vi "read_Shapes.vi"() -> ()   [LabVIEW 2019]
uses:
  Program Files (x86)/National Instruments/LabVIEW 2019/examples/RTI DDS Toolkit/ShapesDemo/support/RTI Connext DDS Shape Type.ctl
  <vilib>/RTI DDS Toolkit/Types/DDS Sample Info.ctl
  <vilib>/RTI DDS Toolkit/Types/RTI DDS Advanced Reader Configuration.ctl
  <vilib>/RTI DDS Toolkit/Library/LVDDS_library.lvlib
panel:
  in  "Tab Control":enum32{"Main", "config"}(tab)
  out "DDS Data":string[][](table)=[["RED", "203", "241", " 30"]]
  in  "Query condition":string
  out "Sample Info":T1={"DDS_SampleStateKind"=enum."DDS_NOT_READ_SAMPLE_STATE", "DDS_ViewStateKind"=enum."DDS_NOT_NEW_VIEW_STATE", "DDS_InstanceStateKind"=enum."DDS_ALIVE_INSTANCE_STATE", "sec"=1653553695, "nanosec"=521993280, "valid_data"=TRUE}
  out "XY Graph":cluster{"Y":dbl[], "Y":dbl[]}[](graph)=[{"Y"=[203.0], "Y"=[241.0]}]
  out "shapesize":i32(slide)=30 scale=0.0..100.0
  in  "Enter a shape 'color' to see the square moving in 'XY Graph' and its size in 'shapesize'":string="RED"
  in  "Enable DDS":bool=TRUE
  in  "Stop":bool
  in  "Type Name":string="ShapeType"
  in  "Key Name":string="color"
  in  "Topic Name":string="Circle"
  in  "Advanced Reader Configuration":T2
  in  "error in (no error)":errorcluster
  in  "ShapeType 2":T3
  out "error out":errorcluster
  out "ShapeType":T3={"color"="RED", "x"=203, "y"=241, "shapesize"=30}
  # "RTI DDS Read shape"
  # "Source Timestamp"
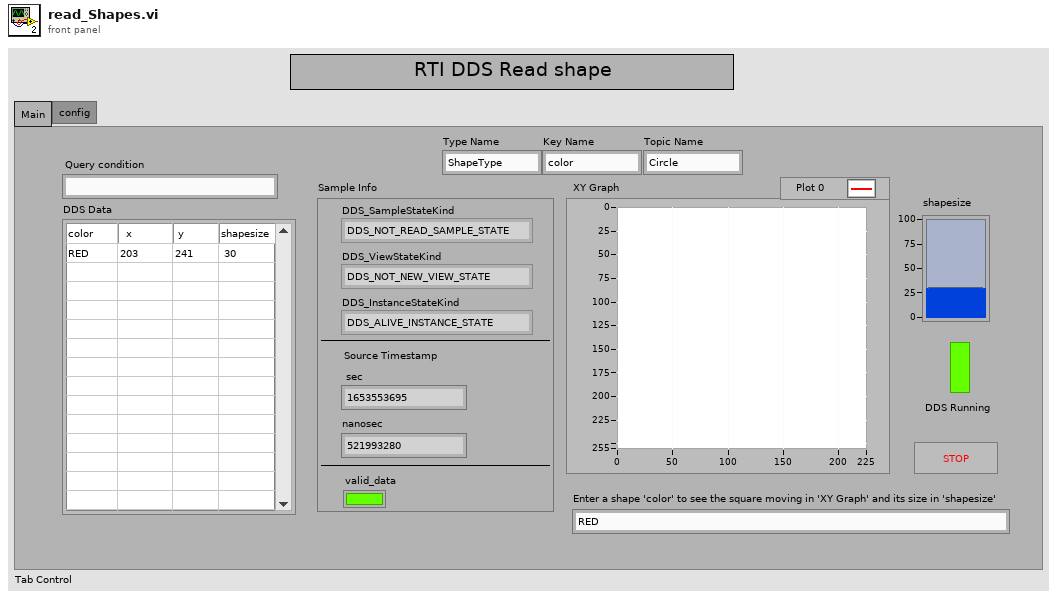
[diagram p1: front panel]
types:
  T1 = typedef "LVDDS_library.lvlib/DDS Sample Info.ctl" = cluster{"DDS_SampleStateKind":enum32{"DDS_INVALID_SAMPLE_STATE", "DDS_READ_SAMPLE_STATE", "DDS_NOT_READ_SAMPLE_STATE"}, "DDS_ViewStateKind":enum32{"DDS_INVALID_SAMPLE_STATE", "DDS_NEW_VIEW_STATE", "DDS_NOT_NEW_VIEW_STATE"}, "DDS_InstanceStateKind":enum32{"DDS_INVALID_STATE", "DDS_ALIVE_INSTANCE_STATE", "DDS_NOT_ALIVE_DISPOSED_INSTANCE_STATE", "", "DDS_NOT_ALIVE_NO_WRITERS_INSTANCE_STATE"}, "sec":i32, "nanosec":u32, "valid_data":bool}
  T2 = typedef "LVDDS_library.lvlib/RTI DDS Advanced Reader Configuration.ctl" = cluster{"typeName":string, "keyName":string, "domainParticipantQoSProfile":string, "dataReaderQoSProfile":string, "forceArrayMapping?":bool, "forceExclusiveReader?":bool, "forceRead? (only ExclusiveReader)":bool, "forceUnboundedString?":bool}
  T3 = typedef "RTI Connext DDS Shape Type.ctl" = cluster{"color":string, "x":i32, "y":i32, "shapesize":i32}
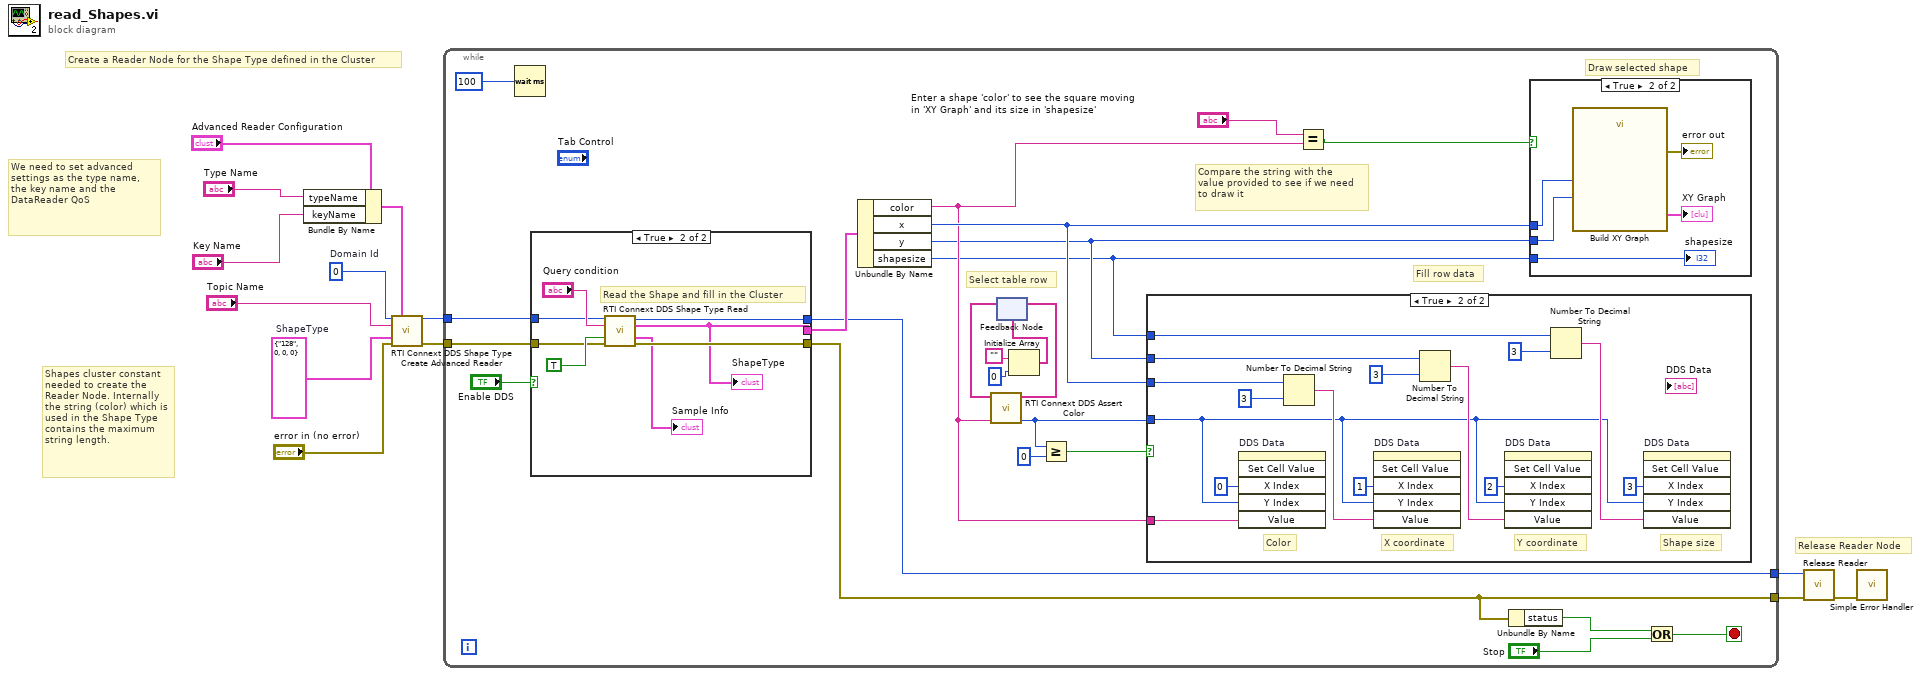
[diagram p0: block diagram]
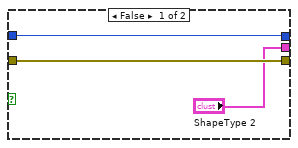
[diagram p3: hidden frame]
diagram:
  w7 = T3 {"color"="128", "x"=0, "y"=0, "shapesize"=0}  # ShapeType
  w2 = u32 0  # Domain Id
  # "We need to set advanced settings as the type name,\nthe key name and the DataReader QoS"
  # "Release Reader Node"
  # "Shapes cluster constant needed to create the Reader Node. Internally the string (color) which is used in the Shape Type contains the maximum string length."
  # "Create a Reader Node for the Shape Type defined in the Cluster"
  n1 = Bundle By Name(cluster="Advanced Reader Configuration", "typeName"="Type Name", "keyName"="Key Name") -> (w6:T2)
  n2 = call "RTI Connext DDS Shape Type Create Advanced Reader.vi"("Domain Id"=w2, "Advanced Reader Configuration"=w6, "Topic Name"="Topic Name", "MyComplexType type"=w7, "error in (no error)"="error in (no error)") -> ("DDS Object Ref"=w1:u64, "error out"=w5:errorcluster)  [unwired: 9 in]
  n3 = while {
    tunnel: [w15] -> w13
    tunnel: w5 -> [w21]
    tunnel: [w20] -> w4
    tunnel: w1 -> [w14]
    stop <- w26 stop-if-true
    # "Compare the string with the\nvalue provided to see if we need\nto draw it"
    # "Select table row"
    # "Draw selected shape"
    # "Fill row data"
    n4 = Wait (ms)(milliseconds to wait=u32 100) -> ()  [unwired: 1 out]
    n5 = case shown="True" "Enable DDS" {
      tunnel: ["ShapeType 2" w56] -> w36
      tunnel: w14 -> [w55 w59]
      tunnel: w21 -> [w54 w58]
      tunnel: [w55 w57] -> w15
      tunnel: [w54 w63] -> w20
      frame False {
      }
      frame True {
        # "Read the Shape and fill in the Cluster"
        n6 = call "RTI Connext DDS Shape Type Read.vi"("DDS Object Ref in"=w59, "Query Condition"="Query condition", "Only New Samples"=TRUE, "error in (no error)"=w58) -> ("DDS Object Ref out"=w57:u64, "Read Sample"=w56:T3, "DDS Sample Info"=→"Sample Info":T1, "error out"=w63:errorcluster)  [unwired: 7 in, 1 out]
        "ShapeType" <- w56
      }
    }
    n7 = Unbundle By Name(w36) -> ("color"=w22:string, "x"=w37:i32, "y"=w17:i32, "shapesize"=w16:i32)
    n8 = Initialize Array("", 0 ("dimension size")) -> (w33:string[])
    n9 = feedback #1(w33) -> (w28:string[])
    n10 = call "RTI Connext DDS Assert Color.vi"("Color"=w22, "Input Array"=w28) -> ("Position"=w18:i32, "Output Array"=w29:string[])  [unwired: 8 in]
    n11 = feedback-in #1(w29) -> ()
    n12 = Greater Or Equal?(x=w18, y=0) -> (x >= y?=w32:bool)
    n13 = case shown="True" w32 {
      tunnel: w37 -> [_ w51]
      tunnel: w17 -> [_ w50]
      tunnel: w18 -> [_ w39]
      tunnel: w22 -> [_ w46]
      tunnel: w16 -> [_ w49]
      frame False {
      }
      frame True {
        # "Shape size"
        # "Y coordinate"
        # "X coordinate"
        # "Color"
        n14 = invoke on="DDS Data" class="Tbl (strict)" method="Set Cell Value"("X Index"=0, "Y Index"=w39, "Value"=w46) -> ()  [unwired: 3 in, 6 out]
        n15 = Number To Decimal String(number=w51, width (-)=3) -> (decimal integer string=w43:string)
        n16 = invoke on="DDS Data" class="Tbl (strict)" method="Set Cell Value"("X Index"=1, "Y Index"=w39, "Value"=w43) -> ()  [unwired: 3 in, 6 out]
        n17 = Number To Decimal String(number=w50, width (-)=3) -> (decimal integer string=w42:string)
        n18 = invoke on="DDS Data" class="Tbl (strict)" method="Set Cell Value"("X Index"=2, "Y Index"=w39, "Value"=w42) -> ()  [unwired: 3 in, 6 out]
        n19 = Number To Decimal String(number=w49, width (-)=3) -> (decimal integer string=w40:string)
        n20 = invoke on="DDS Data" class="Tbl (strict)" method="Set Cell Value"("X Index"=3, "Y Index"=w39, "Value"=w40) -> ()  [unwired: 3 in, 6 out]
      }
    }
    n21 = Equal?(x="Enter a shape 'color' to see the square moving in 'XY Graph' and its size in 'shapesize'", y=w22) -> (x = y?=w24:bool)
    n22 = Unbundle By Name(w20) -> ("status"=w19:bool)
    n23 = case shown="True" w24 {
      tunnel: w37 -> [_ w65]
      tunnel: w17 -> [_ w67]
      tunnel: w16 -> [_ w66]
      frame False {
      }
      frame True {
        n24 = call "Build XY Graph"("Y Input"=w67, "X Input"=w65) -> ("error out"=→"error out":errorcluster, "XY Graph"=→"XY Graph":cluster{"Y":dbl[], "Y":dbl[]}[])  [unwired: 3 in, 5 out]
        "shapesize" <- w66
      }
    }
    n25 = Or(x=w19, y="Stop") -> (x .or. y?=w26:bool)
  }
  n26 = call <vilib>:"Release Reader.vi"("error in (no error)"=w4, "DDS Object Ref"=w13) -> ("error out"=w12:errorcluster)  [unwired: 9 in]
  n27 = call <vilib>:"Simple Error Handler.vi"("error in (no error)"=w12) -> ()  [unwired: 4 in, 5 out]
